vi "Main.vi"(7 "sweep rate, /min":dbl=0.2, 8 "sweep to:":dbl=-0.5, 9 "sweep":T6(radio)=enum."time_sweep") -> ()   [LabVIEW 2017] (continued)
                    n4522 = property on="Down Rate" class="DigNum (strict)"() -> ("Value"=w5909:dbl)  [unwired: 2 in, 2 out]
                    n4523 = property on="lower limit" class="DigNum (strict)"() -> ("Value"=w5910:dbl)  [unwired: 2 in, 2 out]
                    n4524 = property on="sweep to:" class="DigNum (strict)"("Value"=w5910) -> ()  [unwired: 2 in, 2 out]
                    n4525 = property on="sweep rate, /min" class="DigNum (strict)"("Value"=w5909) -> ()  [unwired: 2 in, 2 out]
                  }
                  frame "Sweep Up" {
                    n4526 = property on="Up Rate" class="DigNum (strict)"() -> ("Value"=w5911:dbl)  [unwired: 2 in, 2 out]
                    n4527 = property on="upper limit" class="DigNum (strict)"() -> ("Value"=w5912:dbl)  [unwired: 2 in, 2 out]
                    n4528 = property on="sweep to:" class="DigNum (strict)"("Value"=w5912) -> ()  [unwired: 2 in, 2 out]
                    n4529 = property on="sweep rate, /min" class="DigNum (strict)"("Value"=w5911) -> ()  [unwired: 2 in, 2 out]
                  }
                  frame "True" {
                  }
                }
              }
              frame #3 {
                n4530 = Enqueue Element(queue=w5914, element="Start Sweep") -> ()  [unwired: 2 in, 3 out]
              }
            }
          }
          frame True {
            # "When step values are all finished"
            n4531 = property on="HyperLoop" class="Bool (strict)"() -> ("Value"=w5916:bool)  [unwired: 2 in, 2 out]
            n4532 = property on="Table Index" class="DigNum (strict)"("Value"=0.0 ("Table Index")) -> ()  [unwired: 2 in, 2 out]
            n4533 = case shown="True" w5916 {
              tunnel: w5917 -> [w5923 w5928]
              frame False {
                n4534 = Enqueue Element(queue=w5923, element="Idle") -> ()  [unwired: 2 in, 3 out]
                n4535 = property on="Start Mapping" class="Bool"("DisabledEnum"=T12."Enabled" ("Disabled")) -> ()  [unwired: 2 in, 2 out]
                n4536 = property on="Stop Mapping" class="Bool"("DisabledEnum"=T12."Disabled and Grayed Out" ("Disabled")) -> ()  [unwired: 2 in, 2 out]
                n4537 = property on="Sweep Direction" class="Str"("Value"="Finished!" ("Sweep Direction"), "Text.TextColor"=u32 16711680 ("Text.Text Colors:Text Color")) -> ()  [unwired: 2 in, 2 out]
              }
              frame True {
                n4538 = Enqueue Element(queue=w5928, element="Step to Next HyperLoop Value") -> ()  [unwired: 2 in, 3 out]
                n4539 = property on="HyperLoop Index" class="DigNum (strict)"() -> ("Value"=w5926:dbl)  [unwired: 2 in, 2 out]
                n4540 = property on="Start Mapping" class="Bool"("DisabledEnum"=T12."Enabled" ("Disabled")) -> ()  [unwired: 2 in, 2 out]
                n4541 = property on="Stop Mapping" class="Bool"("DisabledEnum"=T12."Disabled and Grayed Out" ("Disabled")) -> ()  [unwired: 2 in, 2 out]
                n4542 = Increment(x=w5926) -> (x+1=w5927:dbl)
                n4543 = property on="HyperLoop Index" class="DigNum (strict)"("Value"=w5927) -> ()  [unwired: 2 in, 2 out]
                n4544 = property on="Sweep Direction" class="Str"("Value"="Finished!" ("Sweep Direction"), "Text.TextColor"=u32 16711680 ("Text.Text Colors:Text Color")) -> ()  [unwired: 2 in, 2 out]
              }
            }
          }
        }
      }
      frame "Step to Next HyperLoop Value" {
        n4545 = property on="HyperLoop Index" class="DigNum (strict)"() -> ("Value"=w5933:dbl)  [unwired: 2 in, 2 out]
        n4546 = property on="HyperLoop Steps" class="Tbl (strict)"() -> ("Value"=w5932:string[][])  [unwired: 2 in, 2 out]
        n4547 = Equal?(x=w5933, y=0) -> (x = y?=w5944:bool)
        n4548 = case shown="True" w5944 {
          tunnel: w5933 -> [w5952 w5958]
          tunnel: cluster{"Row":i32, "Column":i32} {"Row"=0, "Column"=0} ("Active Cell:Active Cell") -> [w5951 w5957]
          frame False {
            w5953 = 0 ("Column")
            n4549 = Decrement(x=w5952) -> (x-1=w5954:dbl)
            n4550 = Bundle By Name(cluster=w5951, "Row"=w5952, "Column"=w5953) -> (w5950:cluster{"Row":i32, "Column":i32})
            n4551 = Bundle By Name(cluster=w5950, "Row"=w5954, "Column"=w5953) -> (w5948:cluster{"Row":i32, "Column":i32})
            n4552 = property on="HyperLoop Steps" class="Tbl (strict)"("Active Cell"=w5948, "Cell BG Color"=u32 16711680 ("Active Cell:Cell Background Color")) -> ()  [unwired: 2 in, 2 out]
            n4553 = property on="HyperLoop Steps" class="Tbl (strict)"("Active Cell"=w5950, "Cell BG Color"=u32 16776072 ("Active Cell:Cell Background Color")) -> ()  [unwired: 2 in, 2 out]
          }
          frame True {
            n4554 = Bundle By Name(cluster=w5957, "Row"=w5958, "Column"=0) -> (w5956:cluster{"Row":i32, "Column":i32})
            n4555 = property on="HyperLoop Steps" class="Tbl (strict)"("Active Cell"=w5956, "Cell BG Color"=u32 16776072 ("Active Cell:Cell Background Color")) -> ()  [unwired: 2 in, 2 out]
          }
        }
        n4556 = call <vilib>:"Space Constant.vi"() -> ("String"=w5942:string)
        n4557 = Index Array(array=w5932, index (row)=w5933, index (col)=0 ("disabled index (col)")) -> (element=w5941:string)
        n4558 = call <vilib>:"Search and Replace Pattern.vi"("string"=w5941, "regular expression (\"\")"=w5942, "replace string (\"\")"="" ("replace string (\"\")"), "replace all? (F)"=TRUE) -> ("result string"=w5945:string)  [unwired: 1 in, 1 out]
        n4559 = Equal?(x="", y=w5945) -> (x = y?=w5943:bool)
        n4560 = Fract/Exp String To Number(string=w5945) -> (number=w5946:dbl)  [unwired: 3 in, 1 out]
        n4561 = case shown="False" w5943 {
          tunnel: w5946 -> [w5960 _]
          tunnel: w5935 -> [w5961 w6137]
          frame False {
            # "When step values are not finished"
            n4562 = stacked-sequence {
              tunnel: w5960 -> [w5963 _ _]
              tunnel: w5961 -> [_ _ _]
              frame #0 {
                # "1 = 2400 1\n2 = 2400 2\n\n4 = 2636a smua\n5 = 2636a smub\n6 = do not sweep, just time\n7 = iPS, magnetic field \n8 = iTC, temperature"
                # "set next value in the sweep"
                n4563 = property on="step_hyper" class="RadioBtnsControl (strict)"() -> ("Value"=w5962:T9)  [unwired: 2 in, 2 out]
                n4564 = case shown="\"iTC_HyperLoop\"" w5962 {
                  tunnel: w5963 -> [w5965 w5972 _ _ _ w6030 w6094]
                  tunnel: w5963 -> [_ _ w5981 w6007 _ _ _]
                  frame "2400_1_HyperLoop" {
                    # "sweep voltage on 2400 1"
                    n4565 = property on="2400_1_addr_hyper" class="DigNum (strict)"() -> ("Value"=w5964:u8)  [unwired: 2 in, 2 out]
                    n4566 = Number To Fractional String(number=w5965) -> (F-format string=w5970:string)  [unwired: 3 in]
                    n4567 = Concatenate Strings(":INIT:IMM; :SOUR:VOLT:LEV:IMM:AMPL " ("data"), w5970) -> (w5968:string)
                    n4568 = Number To Decimal String(number=w5964) -> (decimal integer string=w5966:string)  [unwired: 1 in]
                    n4569 = GPIB Write(0:w5966, 1:w5968, 2:i16 1 ("mode (0)")) -> ()  [unwired: 2 in, 2 out]
                  }
                  frame "2400_2_HyperLoop" {
                    # "sweep voltage on 2400 2"
                    n4570 = property on="2400_2_addr_hyper" class="DigNum (strict)"() -> ("Value"=w5971:u8)  [unwired: 2 in, 2 out]
                    n4571 = Number To Fractional String(number=w5972) -> (F-format string=w5977:string)  [unwired: 3 in]
                    n4572 = Concatenate Strings(":INIT:IMM; :SOUR:CURR:LEV:IMM:AMPL " ("data"), w5977) -> (w5975:string)
                    n4573 = Number To Decimal String(number=w5971) -> (decimal integer string=w5973:string)  [unwired: 1 in]
                    n4574 = GPIB Write(0:w5973, 1:w5975, 2:i16 1 ("mode (0)")) -> ()  [unwired: 2 in, 2 out]
                  }
                  frame "2636_smua_HyperLoop" {
                    # "sweep voltage on 2636a smua"
                    n4575 = property on="Hyper Channel" class="DigNum (strict)"() -> ("Value"=w5978:dbl)  [unwired: 2 in, 2 out]
                    n4576 = property on="2336A_addr_hyper" class="VISAName"() -> ("Value"=w5979:refnum<visa-resource-name>)  [unwired: 2 in, 2 out]
                    n4577 = property on="Hyper_Mini steps" class="DigNum (strict)"() -> ("Value"=w5980:dbl)  [unwired: 2 in, 2 out]
                    n4578 = Subtract(x=w5981, y=w5978) -> (x-y=w5982:dbl)
                    n4579 = Divide(x=w5982, y=w5980) -> (x/y=w5983:dbl)
                    n4580 = for {
                      N: w5980 -> [_]
                      tunnel: w5978 -> [w5993]
                      tunnel: w5983 -> [w5992]
                      tunnel: w5979 -> [w5989]
                      i -> [w5988]
                      n4581 = Increment(x=w5988) -> (x+1=w5987:i32)
                      n4582 = Multiply(x=w5992, y=w5987) -> (x*y=w5991:dbl)
                      n4583 = Add(x=w5991, y=w5993) -> (x+y=w5984:dbl)
                      n4584 = call "setLevel.vi"("VISA resource name 2"=w5989, "Source"=Source."Voltage", "Channel"=Channel."a", "SourceLevel"=w5984) -> ("VISA resource name"=w5986:refnum<visa-resource-name>)  [unwired: 1 in, 2 out]
                      n4585 = Wait (ms)(milliseconds to wait=u32 12) -> ()  [unwired: 1 out]
                      n4586 = property on="diagonal_hyper" class="Bool (strict)"() -> ("Value"=w5985:bool)  [unwired: 2 in, 2 out]
                      n4587 = property on="Hyper Channel" class="DigNum (strict)"("Value"=w5984) -> ()  [unwired: 2 in, 2 out]
                      n4588 = case shown="True" w5985 {
                        tunnel: w5984 -> [_ w6003]
                        tunnel: w5986 -> [_ w5998]
                        frame False {
                        }
                        frame True {
                          n4589 = property on="Hyper Offset" class="DigNum (strict)"() -> ("Value"=w5996:dbl)  [unwired: 2 in, 2 out]
                          n4590 = property on="Hyper Slope" class="DigNum (strict)"() -> ("Value"=w5997:dbl)  [unwired: 2 in, 2 out]
                          n4591 = Multiply(x=w6003, y=w5997) -> (x*y=w6002:dbl)
                          n4592 = Add(x=w6002, y=w5996) -> (x+y=w5999:dbl)
                          n4593 = call "setLevel.vi"("VISA resource name 2"=w5998, "Source"=Source."Voltage", "Channel"=Channel."b", "SourceLevel"=w5999) -> ()  [unwired: 1 in, 3 out]
                        }
                      }
                    }
                  }
                  frame "2636_smub_HyperLoop" {
                    # "sweep voltage on 2636a smua"
                    n4594 = property on="Hyper Channel" class="DigNum (strict)"() -> ("Value"=w6004:dbl)  [unwired: 2 in, 2 out]
                    n4595 = property on="Hyper_Mini steps" class="DigNum (strict)"() -> ("Value"=w6006:dbl)  [unwired: 2 in, 2 out]
                    n4596 = property on="2336A_addr_hyper" class="VISAName"() -> ("Value"=w6005:refnum<visa-resource-name>)  [unwired: 2 in, 2 out]
                    n4597 = Subtract(x=w6007, y=w6004) -> (x-y=w6008:dbl)
                    n4598 = Divide(x=w6008, y=w6006) -> (x/y=w6009:dbl)
                    n4599 = for {
                      N: w6006 -> [_]
                      tunnel: w6004 -> [w6019]
                      tunnel: w6009 -> [w6018]
                      tunnel: w6005 -> [w6015]
                      i -> [w6014]
                      n4600 = Increment(x=w6014) -> (x+1=w6013:i32)
                      n4601 = Multiply(x=w6018, y=w6013) -> (x*y=w6017:dbl)
                      n4602 = Add(x=w6017, y=w6019) -> (x+y=w6010:dbl)
                      n4603 = property on="diagonal_hyper" class="Bool (strict)"() -> ("Value"=w6011:bool)  [unwired: 2 in, 2 out]
                      n4604 = call "setLevel.vi"("VISA resource name 2"=w6015, "Source"=Source."Voltage", "Channel"=Channel."b", "SourceLevel"=w6010) -> ("VISA resource name"=w6012:refnum<visa-resource-name>)  [unwired: 1 in, 2 out]
                      n4605 = Wait (ms)(milliseconds to wait=u32 12) -> ()  [unwired: 1 out]
                      n4606 = case shown="True" w6011 {
                        tunnel: w6010 -> [_ w6029]
                        tunnel: w6012 -> [_ w6024]
                        frame False {
                        }
                        frame True {
                          n4607 = property on="Hyper Offset" class="DigNum (strict)"() -> ("Value"=w6022:dbl)  [unwired: 2 in, 2 out]
                          n4608 = property on="Hyper Slope" class="DigNum (strict)"() -> ("Value"=w6023:dbl)  [unwired: 2 in, 2 out]
                          n4609 = Multiply(x=w6029, y=w6023) -> (x*y=w6028:dbl)
                          n4610 = Add(x=w6028, y=w6022) -> (x+y=w6025:dbl)
                          n4611 = call "setLevel.vi"("VISA resource name 2"=w6024, "Source"=Source."Voltage", "Channel"=Channel."a", "SourceLevel"=w6025) -> ()  [unwired: 1 in, 3 out]
                        }
                      }
                      n4612 = property on="Hyper Channel" class="DigNum (strict)"("Value"=w6010) -> ()  [unwired: 2 in, 2 out]
                    }
                  }
                  frame "time_HyperLoop", Default {
                    # "do not sweep, just time"
                  }
                  frame "iPS_HyperLoop" {
                    # "step magnetic field"
                    n4613 = stacked-sequence {
                      tunnel: w6030 -> [_ _ _ _ w6045 _ _ _ w6057 _ w6060 _]
                      frame #0 {
                        n4614 = property on="HyperLoop Index" class="DigNum (strict)"() -> ("Value"=w6031:dbl)  [unwired: 2 in, 2 out]
                        n4615 = Equal?(x=w6031, y=0.0) -> (x = y?=w6032:bool)
                        n4616 = case shown="True" w6032 {
                          frame False {
                          }
                          frame True {
                            n4617 = property on="iPS _addr_hyper" class="VISAName"() -> ("Value"=w6036:refnum<visa-resource-name>)  [unwired: 2 in, 2 out]
                            n4618 = property on="Hyper_FieldRate\n(T/min)" class="DigNum (strict)"() -> ("Value"=w6034:dbl)  [unwired: 2 in, 2 out]
                            n4619 = call "iPSset.vi"("Field Rate, T/min"=w6034, "iPSSetCtrl"=iPSsetCtrl."Set Target Field Rate", "VISA resource name"=w6036) -> ("VISA resource name out"=w6035:refnum<visa-resource-name>)  [unwired: 5 in, 3 out]
                            n4620 = property on="iPS _addr_hyper" class="VISAName"("Value"=w6035) -> ()  [unwired: 2 in, 2 out]
                          }
                        }
                      }
                      frame #1 {
                        n4621 = Wait (ms)(milliseconds to wait=u32 500) -> ()  [unwired: 1 out]
                      }
                      frame #2 {
                        n4622 = property on="iPS _addr_hyper" class="VISAName"() -> ("Value"=w6039:refnum<visa-resource-name>)  [unwired: 2 in, 2 out]
                        n4623 = call "iPSset.vi"("iPSSetCtrl"=iPSsetCtrl."Hold", "VISA resource name"=w6039) -> ("VISA resource name out"=w6040:refnum<visa-resource-name>)  [unwired: 6 in, 3 out]
                        n4624 = property on="iPS _addr_hyper" class="VISAName"("Value"=w6040) -> ()  [unwired: 2 in, 2 out]
                      }
                      frame #3 {
                        n4625 = Wait (ms)(milliseconds to wait=u32 500) -> ()  [unwired: 1 out]
                      }
                      frame #4 {
                        n4626 = property on="iPS _addr_hyper" class="VISAName"() -> ("Value"=w6043:refnum<visa-resource-name>)  [unwired: 2 in, 2 out]
                        n4627 = call "iPSset.vi"("Target Field, T"=w6045, "iPSSetCtrl"=iPSsetCtrl."Set Target Field", "VISA resource name"=w6043) -> ("VISA resource name out"=w6044:refnum<visa-resource-name>)  [unwired: 5 in, 3 out]
                        n4628 = property on="iPS _addr_hyper" class="VISAName"("Value"=w6044) -> ()  [unwired: 2 in, 2 out]
                      }
                      frame #5 {
                        n4629 = Wait (ms)(milliseconds to wait=u32 500) -> ()  [unwired: 1 out]
                      }
                      frame #6 {
                        n4630 = property on="iPS _addr_hyper" class="VISAName"() -> ("Value"=w6048:refnum<visa-resource-name>)  [unwired: 2 in, 2 out]
                        n4631 = call "iPSset.vi"("iPSSetCtrl"=iPSsetCtrl."Hold", "VISA resource name"=w6048) -> ("VISA resource name out"=w6049:refnum<visa-resource-name>)  [unwired: 6 in, 3 out]
                        n4632 = property on="iPS _addr_hyper" class="VISAName"("Value"=w6049) -> ()  [unwired: 2 in, 2 out]
                      }
                      frame #7 {
                        n4633 = Wait (ms)(milliseconds to wait=u32 500) -> ()  [unwired: 1 out]
                      }
                      frame #8 {
                        n4634 = Equal To 0?(x=w6057) -> (x = 0?=w6056:bool)
                        n4635 = property on="iPS _addr_hyper" class="VISAName"() -> ("Value"=w6052:refnum<visa-resource-name>)  [unwired: 2 in, 2 out]
                        n4636 = Select(t=iPSsetCtrl."Go to Zero" ("iPSSetCtrl"), s=w6056, f=iPSsetCtrl."Go to Field" ("iPSSetCtrl")) -> (s? t:f=w6053:T18)
                        n4637 = call "iPSset.vi"("iPSSetCtrl"=w6053, "VISA resource name"=w6052) -> ()  [unwired: 6 in, 4 out]
                      }
                      frame #9 {
                        n4638 = Wait (ms)(milliseconds to wait=u32 500) -> ()  [unwired: 1 out]
                      }
                      frame #10 {
                        n4639 = while {
                          tunnel: w6060 -> [w6091]
                          stop <- w6087 stop-if-true
                          n4640 = property on="iPS _addr_hyper" class="VISAName"() -> ("Value"=w6086:refnum<visa-resource-name>)  [unwired: 2 in, 2 out]
                          n4641 = call "iPSread.vi"("iPSreadCtrl"=iPSreadCtrl."MagnetField", "VISA resource name"=w6086) -> ("number"=w6083:dbl, "VISA resource name out"=w6085:refnum<visa-resource-name>)  [unwired: 6 in, 2 out]
                          n4642 = property on="Tolerance_Hyper" class="DigNum (strict)"() -> ("Value"=w6084:dbl)  [unwired: 2 in, 2 out]
                          n4643 = property on="iPS _addr_hyper" class="VISAName"("Value"=w6085) -> ()  [unwired: 2 in, 2 out]
                          n4644 = Wait (ms)(milliseconds to wait=u32 500) -> ()  [unwired: 1 out]
                          n4645 = Subtract(x=w6083, y=w6091) -> (x-y=w6090:dbl)
                          n4646 = Absolute Value(x=w6090) -> (abs(x)=w6089:dbl)
                          n4647 = Less Or Equal?(x=w6089, y=w6084) -> (x <= y?=w6087:bool)
                          n4648 = property on="Hyper Channel" class="DigNum (strict)"("Value"=w6083) -> ()  [unwired: 2 in, 2 out]
                          n4649 = property on="at field_hyper" class="Bool (strict)"("Value"=w6087) -> ()  [unwired: 2 in, 2 out]
                        }
                        n4650 = property on="diagonal_hyper" class="Bool (strict)"() -> ("Value"=w6059:bool)  [unwired: 2 in, 2 out]
                        n4651 = case shown="True" w6059 {
                          tunnel: w6060 -> [_ w6068]
                          frame False {
                          }
                          frame True {
                            n4652 = property on="Channel hyper" class="Enum (strict)"() -> ("Value"=w6062:T2)  [unwired: 2 in, 2 out]
                            n4653 = property on="2336A_addr_hyper" class="VISAName"() -> ("Value"=w6061:refnum<visa-resource-name>)  [unwired: 2 in, 2 out]
                            n4654 = property on="Hyper Offset" class="DigNum (strict)"() -> ("Value"=w6064:dbl)  [unwired: 2 in, 2 out]
                            n4655 = property on="Hyper Slope" class="DigNum (strict)"() -> ("Value"=w6065:dbl)  [unwired: 2 in, 2 out]
                            n4656 = call "SinglePointMeasurement.vi"("Measure"=Measure."Voltage", "Channel"=w6062, "VISA resource name 2"=w6061) -> ("Measuremet"=w6066:dbl)  [unwired: 3 in, 4 out]
                            n4657 = Multiply(x=w6068, y=w6065) -> (x*y=w6072:dbl)
                            n4658 = property on="Hyper_Mini steps" class="DigNum (strict)"() -> ("Value"=w6063:dbl)  [unwired: 2 in, 2 out]
                            n4659 = Add(x=w6072, y=w6064) -> (x+y=w6069:dbl)
                            n4660 = Subtract(x=w6069, y=w6066) -> (x-y=w6070:dbl)
                            n4661 = Divide(x=w6070, y=w6063) -> (x/y=w6071:dbl)
                            n4662 = for {
                              N: w6063 -> [_]
                              tunnel: w6071 -> [w6081]
                              tunnel: w6061 -> [w6078]
                              tunnel: w6066 -> [w6074]
                              i -> [w6076]
                              n4663 = Increment(x=w6076) -> (x+1=w6075:i32)
                              n4664 = Multiply(x=w6081, y=w6075) -> (x*y=w6080:dbl)
                              n4665 = Add(x=w6080, y=w6074) -> (x+y=w6077:dbl)
                              n4666 = property on="Channel 2" class="Enum (strict)"() -> ("Value"=w6073:T2)  [unwired: 2 in, 2 out]
                              n4667 = Wait (ms)(milliseconds to wait=u32 12) -> ()  [unwired: 1 out]
                              n4668 = call "setLevel.vi"("VISA resource name 2"=w6078, "Source"=Source."Voltage", "Channel"=w6073, "SourceLevel"=w6077) -> ()  [unwired: 1 in, 3 out]
                            }
                          }
                        }
                      }
                      frame #11 {
                        n4669 = Wait (ms)(milliseconds to wait=u32 500) -> ()  [unwired: 1 out]
                      }
                    }
                  }
                  frame "iTC_HyperLoop" {
                    # "step temperature"
                    n4670 = stacked-sequence {
                      tunnel: w6094 -> [w6102 w6106 w6112]
                      frame #0 {
                        n4671 = property on="iTC_addr_hyper" class="VISAName"() -> ("Value"=w6096:refnum<visa-resource-name>)  [unwired: 2 in, 2 out]
                        n4672 = Decrement(x=w6102) -> (x-1=w6099:dbl)
                        n4673 = Less Or Equal To 0?(x=w6099) -> (x <= 0?=w6101:bool)
                        n4674 = Select(t=0.0, s=w6101, f=w6099) -> (s? t:f=w6098:dbl)
                        n4675 = call "iTCset.vi"("Set Point"=w6098, "iTCSetCtrl"=iTCsetCtrl."Set VTI Temp", "VISA resource name"=w6096) -> ("VISA resource name out"=w6095:refnum<visa-resource-name>)  [unwired: 5 in, 3 out]
                        n4676 = Wait (ms)(milliseconds to wait=u32 200) -> ()  [unwired: 1 out]
                        n4677 = property on="iTC_addr_hyper" class="VISAName"("Value"=w6095) -> ()  [unwired: 2 in, 2 out]
                      }
                      frame #1 {
                        n4678 = property on="iTC_addr_hyper" class="VISAName"() -> ("Value"=w6104:refnum<visa-resource-name>)  [unwired: 2 in, 2 out]
                        n4679 = Less Or Equal To 0?(x=w6106) -> (x <= 0?=w6110:bool)
                        n4680 = Select(t=0.0, s=w6110, f=w6106) -> (s? t:f=w6108:dbl)
                        n4681 = call "iTCset.vi"("Set Point"=w6108, "iTCSetCtrl"=iTCsetCtrl."Set Sample Temp", "VISA resource name"=w6104) -> ("VISA resource name out"=w6105:refnum<visa-resource-name>)  [unwired: 5 in, 3 out]
                        n4682 = property on="iTC_addr_hyper" class="VISAName"("Value"=w6105) -> ()  [unwired: 2 in, 2 out]
                        n4683 = Wait (ms)(milliseconds to wait=u32 200) -> ()  [unwired: 1 out]
                      }
                      frame #2 {
                        n4684 = while {
                          tunnel: w6112 -> [w6119]
                          stop <- w6115 stop-if-true
                          n4685 = property on="iTC_addr_hyper" class="VISAName"() -> ("Value"=w6116:refnum<visa-resource-name>)  [unwired: 2 in, 2 out]
                          n4686 = property on="Tolerance_Hyper" class="DigNum (strict)"() -> ("Value"=w6114:dbl)  [unwired: 2 in, 2 out]
                          n4687 = call "iTCread.vi"("VISA resource name"=w6116, "iTCreadCtrl"=iTCreadCtrl."Sample Temp") -> ("number"=w6113:dbl)  [unwired: 5 in, 3 out]
                          n4688 = Subtract(x=w6113, y=w6119) -> (x-y=w6118:dbl)
                          n4689 = Absolute Value(x=w6118) -> (abs(x)=w6117:dbl)
                          n4690 = property on="Hyper Channel" class="DigNum (strict)"("Value"=w6113) -> ()  [unwired: 2 in, 2 out]
                          n4691 = Less?(x=w6117, y=w6114) -> (x < y?=w6115:bool)
                          n4692 = property on="at field_hyper" class="Bool (strict)"("Value"=w6115) -> ()  [unwired: 2 in, 2 out]
                        }
                      }
                    }
                  }
                }
              }
              frame #1 {
                # "Set current hyper channel and wait expected time"
                n4693 = property on="Current Hyper Value" class="DigNum (strict)"() -> ("Value"=w6122:dbl)  [unwired: 2 in, 2 out]
                n4694 = property on="Wait Between Hyper" class="DigNum (strict)"() -> ("Value"=w6121:i32)  [unwired: 2 in, 2 out]
                n4695 = property on="Hyper Channel" class="DigNum (strict)"("Value"=w6122) -> ()  [unwired: 2 in, 2 out]
                n4696 = Multiply(x=w6121, y=1000) -> (x*y=w6123:i32)
                n4697 = Wait (ms)(milliseconds to wait=w6123) -> ()  [unwired: 1 out]
              }
              frame #2 {
                n4698 = stacked-sequence {
                  frame #0 {
                    # "Check if need to swap step direction"
                    n4699 = property on="SwapStepDirection" class="Bool (strict)"() -> ("Value"=w6125:bool)  [unwired: 2 in, 2 out]
                    n4700 = case shown="True" w6125 {
                      frame False {
                      }
                      frame True {
                        n4701 = stacked-sequence {
                          frame #0 {
                            n4702 = property on="HyperLoop Index" class="DigNum (strict)"() -> ("Value"=w6127:dbl)  [unwired: 2 in, 2 out]
                            n4703 = Equal To 0?(x=w6127) -> (x = 0?=w6126:bool)
                            n4704 = case shown="False" w6126 {
                              frame False {
                                n4705 = property on="to" class="DigNum (strict)"() -> ("Value"=w6131:dbl)  [unwired: 2 in, 2 out]
                                n4706 = property on="from" class="DigNum (strict)"() -> ("Value"=w6130:dbl)  [unwired: 2 in, 2 out]
                                n4707 = Swap Values(12:w6131, 14:w6130) -> (1:w6129:dbl, 3:w6128:dbl)  [unwired: 1 in]
                                n4708 = property on="from" class="DigNum (strict)"("Value"=w6128) -> ()  [unwired: 2 in, 2 out]
                                n4709 = property on="to" class="DigNum (strict)"("Value"=w6129) -> ()  [unwired: 2 in, 2 out]
                              }
                              frame True {
                              }
                            }
                          }
                          frame #1 {
                            n4710 = property on="HyperLoop Index" class="DigNum (strict)"() -> ("Value"=w6133:dbl)  [unwired: 2 in, 2 out]
                            n4711 = Equal To 0?(x=w6133) -> (x = 0?=w6132:bool)
                            n4712 = case shown="False" w6132 {
                              frame False {
                                n4713 = property on="Hidden_HyperLoop_Swap" class="Bool (strict)"() -> ("Value"=w6134:bool)  [unwired: 2 in, 2 out]
                                n4714 = property on="Hidden_HyperLoop_Swap" class="Bool (strict)"("Val(Sgnl)"=w6134) -> ()  [unwired: 2 in, 2 out]
                              }
                              frame True {
                              }
                            }
                          }
                        }
                      }
                    }
                  }
                  frame #1 {
                    # "Trigger \"start mapping\" event"
                    n4715 = property on="HyperLoop Hidden" class="Bool (strict)"() -> ("Value"=w6135:bool)  [unwired: 2 in, 2 out]
                    n4716 = property on="HyperLoop Hidden" class="Bool (strict)"("Val(Sgnl)"=w6135) -> ()  [unwired: 2 in, 2 out]
                  }
                }
              }
            }
            n4717 = property on="Current Hyper Value" class="DigNum (strict)"("Value"=w5960) -> ()  [unwired: 2 in, 2 out]
          }
          frame True {
            # "When step values are all finished"
            n4718 = property on="SuperHyper" class="Bool (strict)"() -> ("Value"=w6136:bool)  [unwired: 2 in, 2 out]
            n4719 = case shown="True" w6136 {
              tunnel: w6137 -> [w6143 w6151]
              frame False {
                n4720 = Enqueue Element(queue=w6143, element="Idle") -> ()  [unwired: 2 in, 3 out]
                n4721 = property on="Stop HyperLoop" class="Bool"("DisabledEnum"=T12."Disabled and Grayed Out" ("Disabled")) -> ()  [unwired: 2 in, 2 out]
                n4722 = property on="Start HyperLoop" class="Bool"("DisabledEnum"=T12."Enabled" ("Disabled")) -> ()  [unwired: 2 in, 2 out]
                n4723 = property on="Sweep Direction 2" class="Str"("Value"="Finished!" ("Sweep Direction"), "Text.TextColor"=u32 16711680 ("Text.Text Colors:Text Color")) -> ()  [unwired: 2 in, 2 out]
              }
              frame True {
                n4724 = Enqueue Element(queue=w6151, element="Step to Next SuperHyper Value") -> ()  [unwired: 2 in, 3 out]
                n4725 = property on="SuperHyper_Index" class="DigNum (strict)"() -> ("Value"=w6149:dbl)  [unwired: 2 in, 2 out]
                n4726 = Increment(x=w6149) -> (x+1=w6148:dbl)
                n4727 = property on="Start HyperLoop" class="Bool"("DisabledEnum"=T12."Enabled" ("Disabled")) -> ()  [unwired: 2 in, 2 out]
                n4728 = property on="Stop HyperLoop" class="Bool"("DisabledEnum"=T12."Disabled and Grayed Out" ("Disabled")) -> ()  [unwired: 2 in, 2 out]
                n4729 = property on="SuperHyper_Index" class="DigNum (strict)"("Value"=w6148) -> ()  [unwired: 2 in, 2 out]
                n4730 = property on="Sweep Direction_Hyper" class="Str"("Value"="Finished!" ("Sweep Direction"), "Text.TextColor"=u32 16711680 ("Text.Text Colors:Text Color")) -> ()  [unwired: 2 in, 2 out]
              }
            }
          }
        }
      }
      frame "Step to Next SuperHyper Value" {
        n4731 = property on="SuperHyper_Index" class="DigNum (strict)"() -> ("Value"=w6152:dbl)  [unwired: 2 in, 2 out]
        n4732 = property on="SuperHyper Steps" class="Tbl (strict)"() -> ("Value"=w6153:string[][])  [unwired: 2 in, 2 out]
        n4733 = Equal?(x=w6152, y=0) -> (x = y?=w6164:bool)
        n4734 = case shown="False" w6164 {
          tunnel: w6152 -> [w6172 w6178]
          tunnel: cluster{"Row":i32, "Column":i32} {"Row"=0, "Column"=0} ("Active Cell:Active Cell") -> [w6171 w6177]
          frame False {
            w6173 = 0 ("Column")
            n4735 = Decrement(x=w6172) -> (x-1=w6174:dbl)
            n4736 = Bundle By Name(cluster=w6171, "Row"=w6172, "Column"=w6173) -> (w6170:cluster{"Row":i32, "Column":i32})
            n4737 = Bundle By Name(cluster=w6170, "Row"=w6174, "Column"=w6173) -> (w6168:cluster{"Row":i32, "Column":i32})
            n4738 = property on="SuperHyper Steps" class="Tbl (strict)"("Active Cell"=w6170, "Cell BG Color"=u32 16776072 ("Active Cell:Cell Background Color")) -> ()  [unwired: 2 in, 2 out]
            n4739 = property on="SuperHyper Steps" class="Tbl (strict)"("Active Cell"=w6168, "Cell BG Color"=u32 16711680 ("Active Cell:Cell Background Color")) -> ()  [unwired: 2 in, 2 out]
          }
          frame True {
            n4740 = Bundle By Name(cluster=w6177, "Row"=w6178, "Column"=0) -> (w6176:cluster{"Row":i32, "Column":i32})
            n4741 = property on="SuperHyper Steps" class="Tbl (strict)"("Active Cell"=w6176, "Cell BG Color"=u32 16776072 ("Active Cell:Cell Background Color")) -> ()  [unwired: 2 in, 2 out]
          }
        }
        n4742 = call <vilib>:"Space Constant.vi"() -> ("String"=w6162:string)
        n4743 = Index Array(array=w6153, index (row)=w6152, index (col)=0 ("disabled index (col)")) -> (element=w6161:string)
        n4744 = call <vilib>:"Search and Replace Pattern.vi"("string"=w6161, "regular expression (\"\")"=w6162, "replace string (\"\")"="" ("replace string (\"\")"), "replace all? (F)"=TRUE) -> ("result string"=w6165:string)  [unwired: 1 in, 1 out]
        n4745 = Equal?(x="", y=w6165) -> (x = y?=w6163:bool)
        n4746 = Fract/Exp String To Number(string=w6165) -> (number=w6166:dbl)  [unwired: 3 in, 1 out]
        n4747 = case shown="False" w6163 {
          tunnel: w6166 -> [w6180 _]
          tunnel: w6155 -> [w6181 w6359]
          frame False {
            # "When step values are not finished"
            n4748 = stacked-sequence {
              tunnel: w6180 -> [w6183 _ _ _]
              tunnel: w6181 -> [_ _ _ _]
              frame #0 {
                # "1 = 2400 1\n2 = 2400 2\n\n4 = 2636a smua\n5 = 2636a smub\n6 = do not sweep, just time\n7 = iPS, magnetic field \n8 = iTC, temperature"
                # "set next value in the sweep"
                n4749 = property on="step_super" class="RadioBtnsControl (strict)"() -> ("Value"=w6182:T10)  [unwired: 2 in, 2 out]
                n4750 = case shown="\"2636_smub_SuperHyper\"" w6182 {
                  tunnel: w6183 -> [w6185 w6192 _ _ _ w6250 w6314]
                  tunnel: w6183 -> [_ _ w6201 w6227 _ _ _]
                  frame "2400_1_SuperHyper" {
                    # "sweep voltage on 2400 1"
                    n4751 = property on="2400_1_addr_superhyper" class="DigNum (strict)"() -> ("Value"=w6184:u8)  [unwired: 2 in, 2 out]
                    n4752 = Number To Fractional String(number=w6185) -> (F-format string=w6190:string)  [unwired: 3 in]
                    n4753 = Concatenate Strings(":INIT:IMM; :SOUR:VOLT:LEV:IMM:AMPL " ("data"), w6190) -> (w6188:string)
                    n4754 = Number To Decimal String(number=w6184) -> (decimal integer string=w6186:string)  [unwired: 1 in]
                    n4755 = GPIB Write(0:w6186, 1:w6188, 2:i16 1 ("mode (0)")) -> ()  [unwired: 2 in, 2 out]
                  }
                  frame "2400_2_SuperHyper" {
                    # "sweep voltage on 2400 2"
                    n4756 = property on="2400_2_addr_superhyper" class="DigNum (strict)"() -> ("Value"=w6191:u8)  [unwired: 2 in, 2 out]
                    n4757 = Number To Fractional String(number=w6192) -> (F-format string=w6197:string)  [unwired: 3 in]
                    n4758 = Concatenate Strings(":INIT:IMM; :SOUR:CURR:LEV:IMM:AMPL " ("data"), w6197) -> (w6195:string)
                    n4759 = Number To Decimal String(number=w6191) -> (decimal integer string=w6193:string)  [unwired: 1 in]
                    n4760 = GPIB Write(0:w6193, 1:w6195, 2:i16 1 ("mode (0)")) -> ()  [unwired: 2 in, 2 out]
                  }
                  frame "2636_smua_SuperHyper" {
                    # "sweep voltage on 2636a smua"
                    n4761 = property on="SuperHyper" class="DigNum (strict)"() -> ("Value"=w6198:dbl)  [unwired: 2 in, 2 out]
                    n4762 = property on="Super_ministeps" class="DigNum (strict)"() -> ("Value"=w6199:dbl)  [unwired: 2 in, 2 out]
                    n4763 = property on="2336A_addr_superhyper" class="VISAName"() -> ("Value"=w6200:refnum<visa-resource-name>)  [unwired: 2 in, 2 out]
                    n4764 = Subtract(x=w6201, y=w6198) -> (x-y=w6202:dbl)
                    n4765 = Divide(x=w6202, y=w6199) -> (x/y=w6203:dbl)
                    n4766 = for {
                      N: w6199 -> [_]
                      tunnel: w6198 -> [w6213]
                      tunnel: w6203 -> [w6212]
                      tunnel: w6200 -> [w6209]
                      i -> [w6208]
                      n4767 = Increment(x=w6208) -> (x+1=w6207:i32)
                      n4768 = Multiply(x=w6212, y=w6207) -> (x*y=w6211:dbl)
                      n4769 = Add(x=w6211, y=w6213) -> (x+y=w6204:dbl)
                      n4770 = property on="diagona_super" class="Bool (strict)"() -> ("Value"=w6205:bool)  [unwired: 2 in, 2 out]
                      n4771 = call "setLevel.vi"("VISA resource name 2"=w6209, "Source"=Source."Voltage", "Channel"=Channel."a", "SourceLevel"=w6204) -> ("VISA resource name"=w6206:refnum<visa-resource-name>)  [unwired: 1 in, 2 out]
                      n4772 = Wait (ms)(milliseconds to wait=u32 12) -> ()  [unwired: 1 out]
                      n4773 = case shown="True" w6205 {
                        tunnel: w6204 -> [_ w6223]
                        tunnel: w6206 -> [_ w6218]
                        frame False {
                        }
                        frame True {
                          n4774 = property on="Slope_super" class="DigNum (strict)"() -> ("Value"=w6217:dbl)  [unwired: 2 in, 2 out]
                          n4775 = property on="Offset_super" class="DigNum (strict)"() -> ("Value"=w6216:dbl)  [unwired: 2 in, 2 out]
                          n4776 = Multiply(x=w6223, y=w6217) -> (x*y=w6222:dbl)
                          n4777 = Add(x=w6222, y=w6216) -> (x+y=w6219:dbl)
                          n4778 = call "setLevel.vi"("VISA resource name 2"=w6218, "Source"=Source."Voltage", "Channel"=Channel."b", "SourceLevel"=w6219) -> ()  [unwired: 1 in, 3 out]
                        }
                      }
                      n4779 = property on="SuperHyper" class="DigNum (strict)"("Value"=w6204) -> ()  [unwired: 2 in, 2 out]
                    }
                  }
                  frame "2636_smub_SuperHyper" {
                    # "sweep voltage on 2636a smua"
                    n4780 = property on="SuperHyper" class="DigNum (strict)"() -> ("Value"=w6224:dbl)  [unwired: 2 in, 2 out]
                    n4781 = property on="Super_ministeps" class="DigNum (strict)"() -> ("Value"=w6225:dbl)  [unwired: 2 in, 2 out]
                    n4782 = property on="2336A_addr_superhyper" class="VISAName"() -> ("Value"=w6226:refnum<visa-resource-name>)  [unwired: 2 in, 2 out]
                    n4783 = Subtract(x=w6227, y=w6224) -> (x-y=w6228:dbl)
                    n4784 = Divide(x=w6228, y=w6225) -> (x/y=w6229:dbl)
                    n4785 = for {
                      N: w6225 -> [_]
                      tunnel: w6224 -> [w6239]
                      tunnel: w6229 -> [w6238]
                      tunnel: w6226 -> [w6235]
                      i -> [w6234]
                      n4786 = Increment(x=w6234) -> (x+1=w6233:i32)
                      n4787 = Multiply(x=w6238, y=w6233) -> (x*y=w6237:dbl)
                      n4788 = Add(x=w6237, y=w6239) -> (x+y=w6230:dbl)
                      n4789 = property on="diagona_super" class="Bool (strict)"() -> ("Value"=w6231:bool)  [unwired: 2 in, 2 out]
                      n4790 = call "setLevel.vi"("VISA resource name 2"=w6235, "Source"=Source."Voltage", "Channel"=Channel."b", "SourceLevel"=w6230) -> ("VISA resource name"=w6232:refnum<visa-resource-name>)  [unwired: 1 in, 2 out]
                      n4791 = Wait (ms)(milliseconds to wait=u32 12) -> ()  [unwired: 1 out]
                      n4792 = case shown="True" w6231 {
                        tunnel: w6230 -> [_ w6249]
                        tunnel: w6232 -> [_ w6244]
                        frame False {
                        }
                        frame True {
                          n4793 = property on="Offset_super" class="DigNum (strict)"() -> ("Value"=w6242:dbl)  [unwired: 2 in, 2 out]
                          n4794 = property on="Slope_super" class="DigNum (strict)"() -> ("Value"=w6243:dbl)  [unwired: 2 in, 2 out]
                          n4795 = Multiply(x=w6249, y=w6243) -> (x*y=w6248:dbl)
                          n4796 = Add(x=w6248, y=w6242) -> (x+y=w6245:dbl)
                          n4797 = call "setLevel.vi"("VISA resource name 2"=w6244, "Source"=Source."Voltage", "Channel"=Channel."a", "SourceLevel"=w6245) -> ()  [unwired: 1 in, 3 out]
                        }
                      }
                      n4798 = property on="SuperHyper" class="DigNum (strict)"("Value"=w6230) -> ()  [unwired: 2 in, 2 out]
                    }
                  }
                  frame "time_SuperHyper", Default {
                    # "do not sweep, just time"
                  }
                  frame "iPS_SuperHyper" {
                    # "step magnetic field"
                    n4799 = stacked-sequence {
                      tunnel: w6250 -> [_ _ _ _ w6265 _ _ _ w6277 _ w6280 _]
                      frame #0 {
                        n4800 = property on="SuperHyper_Index" class="DigNum (strict)"() -> ("Value"=w6251:dbl)  [unwired: 2 in, 2 out]
                        n4801 = Equal?(x=w6251, y=0.0) -> (x = y?=w6252:bool)
                        n4802 = case shown="True" w6252 {
                          frame False {
                          }
                          frame True {
                            n4803 = property on="iPS _addr_superhyper" class="VISAName"() -> ("Value"=w6256:refnum<visa-resource-name>)  [unwired: 2 in, 2 out]
                            n4804 = property on="Super_FieldRate\n(T/min)" class="DigNum (strict)"() -> ("Value"=w6255:dbl)  [unwired: 2 in, 2 out]
                            n4805 = call "iPSset.vi"("Field Rate, T/min"=w6255, "iPSSetCtrl"=iPSsetCtrl."Set Target Field Rate", "VISA resource name"=w6256) -> ("VISA resource name out"=w6254:refnum<visa-resource-name>)  [unwired: 5 in, 3 out]
                            n4806 = property on="iPS _addr_superhyper" class="VISAName"("Value"=w6254) -> ()  [unwired: 2 in, 2 out]
                          }
                        }
                      }
                      frame #1 {
                        n4807 = Wait (ms)(milliseconds to wait=u32 500) -> ()  [unwired: 1 out]
                      }
                      frame #2 {
                        n4808 = property on="iPS _addr_superhyper" class="VISAName"() -> ("Value"=w6260:refnum<visa-resource-name>)  [unwired: 2 in, 2 out]
                        n4809 = call "iPSset.vi"("iPSSetCtrl"=iPSsetCtrl."Hold", "VISA resource name"=w6260) -> ("VISA resource name out"=w6259:refnum<visa-resource-name>)  [unwired: 6 in, 3 out]
                        n4810 = property on="iPS _addr_superhyper" class="VISAName"("Value"=w6259) -> ()  [unwired: 2 in, 2 out]
                      }
                      frame #3 {
                        n4811 = Wait (ms)(milliseconds to wait=u32 500) -> ()  [unwired: 1 out]
                      }
                      frame #4 {
                        n4812 = property on="iPS _addr_superhyper" class="VISAName"() -> ("Value"=w6264:refnum<visa-resource-name>)  [unwired: 2 in, 2 out]
                        n4813 = call "iPSset.vi"("Target Field, T"=w6265, "iPSSetCtrl"=iPSsetCtrl."Set Target Field", "VISA resource name"=w6264) -> ("VISA resource name out"=w6263:refnum<visa-resource-name>)  [unwired: 5 in, 3 out]
                        n4814 = property on="iPS _addr_superhyper" class="VISAName"("Value"=w6263) -> ()  [unwired: 2 in, 2 out]
                      }
                      frame #5 {
                        n4815 = Wait (ms)(milliseconds to wait=u32 500) -> ()  [unwired: 1 out]
                      }
                      frame #6 {
                        n4816 = property on="iPS _addr_superhyper" class="VISAName"() -> ("Value"=w6268:refnum<visa-resource-name>)  [unwired: 2 in, 2 out]
                        n4817 = call "iPSset.vi"("iPSSetCtrl"=iPSsetCtrl."Hold", "VISA resource name"=w6268) -> ("VISA resource name out"=w6269:refnum<visa-resource-name>)  [unwired: 6 in, 3 out]
                        n4818 = property on="iPS _addr_superhyper" class="VISAName"("Value"=w6269) -> ()  [unwired: 2 in, 2 out]
                      }
                      frame #7 {
                        n4819 = Wait (ms)(milliseconds to wait=u32 500) -> ()  [unwired: 1 out]
                      }
                      frame #8 {
                        n4820 = Equal To 0?(x=w6277) -> (x = 0?=w6276:bool)
                        n4821 = property on="iPS _addr_superhyper" class="VISAName"() -> ("Value"=w6272:refnum<visa-resource-name>)  [unwired: 2 in, 2 out]
                        n4822 = Select(t=iPSsetCtrl."Go to Zero" ("iPSSetCtrl"), s=w6276, f=iPSsetCtrl."Go to Field" ("iPSSetCtrl")) -> (s? t:f=w6273:T18)
                        n4823 = call "iPSset.vi"("iPSSetCtrl"=w6273, "VISA resource name"=w6272) -> ()  [unwired: 6 in, 4 out]
                      }
                      frame #9 {
                        n4824 = Wait (ms)(milliseconds to wait=u32 500) -> ()  [unwired: 1 out]
                      }
                      frame #10 {
                        n4825 = while {
                          tunnel: w6280 -> [w6311]
                          stop <- w6304 stop-if-true
                          n4826 = property on="iPS _addr_superhyper" class="VISAName"() -> ("Value"=w6307:refnum<visa-resource-name>)  [unwired: 2 in, 2 out]
                          n4827 = call "iPSread.vi"("iPSreadCtrl"=iPSreadCtrl."MagnetField", "VISA resource name"=w6307) -> ("number"=w6305:dbl, "VISA resource name out"=w6306:refnum<visa-resource-name>)  [unwired: 6 in, 2 out]
                          n4828 = property on="Tolerance_super" class="DigNum (strict)"() -> ("Value"=w6303:dbl)  [unwired: 2 in, 2 out]
                          n4829 = Wait (ms)(milliseconds to wait=u32 500) -> ()  [unwired: 1 out]
                          n4830 = Subtract(x=w6305, y=w6311) -> (x-y=w6310:dbl)
                          n4831 = property on="iPS _addr_superhyper" class="VISAName"("Value"=w6306) -> ()  [unwired: 2 in, 2 out]
                          n4832 = Absolute Value(x=w6310) -> (abs(x)=w6309:dbl)
                          n4833 = Less Or Equal?(x=w6309, y=w6303) -> (x <= y?=w6304:bool)
                          n4834 = property on="SuperHyper" class="DigNum (strict)"("Value"=w6305) -> ()  [unwired: 2 in, 2 out]
                          n4835 = property on="at field_super" class="Bool (strict)"("Value"=w6304) -> ()  [unwired: 2 in, 2 out]
                        }
                        n4836 = property on="diagona_super" class="Bool (strict)"() -> ("Value"=w6279:bool)  [unwired: 2 in, 2 out]
                        n4837 = case shown="True" w6279 {
                          tunnel: w6280 -> [_ w6288]
                          frame False {
                          }
                          frame True {
                            n4838 = property on="Channel" class="Enum (strict)"() -> ("Value"=w6281:T2)  [unwired: 2 in, 2 out]
                            n4839 = property on="Offset_super" class="DigNum (strict)"() -> ("Value"=w6284:dbl)  [unwired: 2 in, 2 out]
                            n4840 = property on="2336A_addr_super" class="VISAName"() -> ("Value"=w6282:refnum<visa-resource-name>)  [unwired: 2 in, 2 out]
                            n4841 = property on="Slope_super" class="DigNum (strict)"() -> ("Value"=w6285:dbl)  [unwired: 2 in, 2 out]
                            n4842 = call "SinglePointMeasurement.vi"("Measure"=Measure."Voltage", "Channel"=w6281, "VISA resource name 2"=w6282) -> ("Measuremet"=w6286:dbl)  [unwired: 3 in, 4 out]
                            n4843 = Multiply(x=w6288, y=w6285) -> (x*y=w6292:dbl)
                            n4844 = property on="Super_ministeps" class="DigNum (strict)"() -> ("Value"=w6283:dbl)  [unwired: 2 in, 2 out]
                            n4845 = Add(x=w6292, y=w6284) -> (x+y=w6289:dbl)
                            n4846 = Subtract(x=w6289, y=w6286) -> (x-y=w6290:dbl)
                            n4847 = Divide(x=w6290, y=w6283) -> (x/y=w6291:dbl)
                            n4848 = for {
                              N: w6283 -> [_]
                              tunnel: w6291 -> [w6301]
                              tunnel: w6282 -> [w6298]
                              tunnel: w6286 -> [w6294]
                              i -> [w6296]
                              n4849 = Increment(x=w6296) -> (x+1=w6295:i32)
                              n4850 = Multiply(x=w6301, y=w6295) -> (x*y=w6300:dbl)
                              n4851 = Add(x=w6300, y=w6294) -> (x+y=w6297:dbl)
                              n4852 = property on="Channel 2" class="Enum (strict)"() -> ("Value"=w6293:T2)  [unwired: 2 in, 2 out]
                              n4853 = Wait (ms)(milliseconds to wait=u32 12) -> ()  [unwired: 1 out]
                              n4854 = call "setLevel.vi"("VISA resource name 2"=w6298, "Source"=Source."Voltage", "Channel"=w6293, "SourceLevel"=w6297) -> ()  [unwired: 1 in, 3 out]
                            }
                          }
                        }
                      }
                      frame #11 {
                        n4855 = Wait (ms)(milliseconds to wait=u32 500) -> ()  [unwired: 1 out]
                      }
                    }
                  }
                  frame "iTC_SuperHyper" {
                    # "step temperature"
                    n4856 = stacked-sequence {
                      tunnel: w6314 -> [w6322 w6326 w6332]
                      frame #0 {
                        n4857 = Decrement(x=w6322) -> (x-1=w6319:dbl)
                        n4858 = property on="iTC_addr_super" class="VISAName"() -> ("Value"=w6316:refnum<visa-resource-name>)  [unwired: 2 in, 2 out]
                        n4859 = Less Or Equal To 0?(x=w6319) -> (x <= 0?=w6321:bool)
                        n4860 = Select(t=0.0, s=w6321, f=w6319) -> (s? t:f=w6318:dbl)
                        n4861 = call "iTCset.vi"("Set Point"=w6318, "iTCSetCtrl"=iTCsetCtrl."Set VTI Temp", "VISA resource name"=w6316) -> ("VISA resource name out"=w6315:refnum<visa-resource-name>)  [unwired: 5 in, 3 out]
                        n4862 = Wait (ms)(milliseconds to wait=u32 200) -> ()  [unwired: 1 out]
                        n4863 = property on="iTC_addr_super" class="VISAName"("Value"=w6315) -> ()  [unwired: 2 in, 2 out]
                      }
                      frame #1 {
                        n4864 = property on="iTC_addr_super" class="VISAName"() -> ("Value"=w6325:refnum<visa-resource-name>)  [unwired: 2 in, 2 out]
                        n4865 = Less Or Equal To 0?(x=w6326) -> (x <= 0?=w6330:bool)
                        n4866 = Select(t=0.0, s=w6330, f=w6326) -> (s? t:f=w6328:dbl)
                        n4867 = call "iTCset.vi"("Set Point"=w6328, "iTCSetCtrl"=iTCsetCtrl."Set Sample Temp", "VISA resource name"=w6325) -> ("VISA resource name out"=w6324:refnum<visa-resource-name>)  [unwired: 5 in, 3 out]
                        n4868 = Wait (ms)(milliseconds to wait=u32 200) -> ()  [unwired: 1 out]
                        n4869 = property on="iTC_addr_super" class="VISAName"("Value"=w6324) -> ()  [unwired: 2 in, 2 out]
                      }
                      frame #2 {
                        n4870 = while {
                          tunnel: w6332 -> [w6339]
                          stop <- w6333 stop-if-true
                          n4871 = property on="iTC_addr_super" class="VISAName"() -> ("Value"=w6336:refnum<visa-resource-name>)  [unwired: 2 in, 2 out]
                          n4872 = property on="Tolerance_super" class="DigNum (strict)"() -> ("Value"=w6334:dbl)  [unwired: 2 in, 2 out]
                          n4873 = call "iTCread.vi"("VISA resource name"=w6336, "iTCreadCtrl"=iTCreadCtrl."Sample Temp") -> ("number"=w6335:dbl)  [unwired: 5 in, 3 out]
                          n4874 = Subtract(x=w6335, y=w6339) -> (x-y=w6338:dbl)
                          n4875 = Absolute Value(x=w6338) -> (abs(x)=w6337:dbl)
                          n4876 = property on="SuperHyper" class="DigNum (strict)"("Value"=w6335) -> ()  [unwired: 2 in, 2 out]
                          n4877 = Less?(x=w6337, y=w6334) -> (x < y?=w6333:bool)
                          n4878 = property on="at field_super" class="Bool (strict)"("Value"=w6333) -> ()  [unwired: 2 in, 2 out]
                        }
                      }
                    }
                  }
                }
              }
              frame #1 {
                # "Set current hyper channel and wait expected time"
                n4879 = property on="Current SuperHyper Value" class="DigNum (strict)"() -> ("Value"=w6342:dbl)  [unwired: 2 in, 2 out]
                n4880 = property on="Wait Btwn SuperHyper" class="DigNum (strict)"() -> ("Value"=w6341:i32)  [unwired: 2 in, 2 out]
                n4881 = Multiply(x=w6341, y=1000) -> (x*y=w6343:i32)
                n4882 = property on="SuperHyper" class="DigNum (strict)"("Value"=w6342) -> ()  [unwired: 2 in, 2 out]
                n4883 = Wait (ms)(milliseconds to wait=w6343) -> ()  [unwired: 1 out]
              }
              frame #2 {
                # "Check if need to swap step direction"
                n4884 = property on="SwapHyperDirection" class="Bool (strict)"() -> ("Value"=w6345:bool)  [unwired: 2 in, 2 out]
                n4885 = case shown="True" w6345 {
                  frame False {
                  }
                  frame True {
                    n4886 = stacked-sequence {
                      frame #0 {
                        n4887 = property on="SuperHyper_Index" class="DigNum (strict)"() -> ("Value"=w6346:dbl)  [unwired: 2 in, 2 out]
                        n4888 = Equal To 0?(x=w6346) -> (x = 0?=w6347:bool)
                        n4889 = case shown="False" w6347 {
                          frame False {
                            n4890 = property on="from" class="DigNum (strict)"() -> ("Value"=w6351:dbl)  [unwired: 2 in, 2 out]
                            n4891 = property on="to" class="DigNum (strict)"() -> ("Value"=w6349:dbl)  [unwired: 2 in, 2 out]
                            n4892 = Swap Values(12:w6349, 14:w6351) -> (1:w6348:dbl, 3:w6350:dbl)  [unwired: 1 in]
                            n4893 = property on="from" class="DigNum (strict)"("Value"=w6350) -> ()  [unwired: 2 in, 2 out]
                            n4894 = property on="to" class="DigNum (strict)"("Value"=w6348) -> ()  [unwired: 2 in, 2 out]
                          }
                          frame True {
                          }
                        }
                      }
                      frame #1 {
                        n4895 = property on="Hidden_super_Swap" class="Bool (strict)"() -> ("Value"=w6352:bool)  [unwired: 2 in, 2 out]
                        n4896 = property on="Hidden_super_Swap" class="Bool (strict)"("Val(Sgnl)"=w6352) -> ()  [unwired: 2 in, 2 out]
                      }
                    }
                  }
                }
              }
              frame #3 {
                # "Trigger \"start hyper\" event"
                n4897 = property on="Super Hidden" class="Bool (strict)"() -> ("Value"=w6353:bool)  [unwired: 2 in, 2 out]
                n4898 = property on="Super Hidden" class="Bool (strict)"("Val(Sgnl)"=w6353) -> ()  [unwired: 2 in, 2 out]
              }
            }
            n4899 = property on="Current SuperHyper Value" class="DigNum (strict)"("Value"=w6180) -> ()  [unwired: 2 in, 2 out]
          }
          frame True {
            # "When step values are all finished"
            n4900 = Enqueue Element(queue=w6359, element="Idle") -> ()  [unwired: 2 in, 3 out]
            n4901 = property on="Stop SuperHyper" class="Bool"("DisabledEnum"=T12."Disabled and Grayed Out" ("Disabled")) -> ()  [unwired: 2 in, 2 out]
            n4902 = property on="StartSuperHyper" class="Bool"("DisabledEnum"=T12."Enabled" ("Disabled")) -> ()  [unwired: 2 in, 2 out]
            n4903 = property on="Sweep Direction3" class="Str"("Value"="Finished!" ("Sweep Direction"), "Text.TextColor"=u32 16711680 ("Text.Text Colors:Text Color")) -> ()  [unwired: 2 in, 2 out]
          }
        }
      }
      frame "Quit" {
      }
    }
  }
  n4904 = while {
    tunnel: w3 -> [w6363]
    tunnel: w2 -> [w6361]
    tunnel: w1 -> [w6360]
    stop <- w6362 stop-if-true
    # "This loop is the producer loop."
    n4905 = event shown="[8] \"Populate step table?\": Value Change" {
      selector: _ -> [_ _ _ _ _ _ _ _ _ _ _ _ _ _ _ _ _ _ _ _ _ _ _ _ _ _ _]
      dyn-events: _ -> [_ _ _ _ _ _ _ _ _ _ _ _ _ _ _ _ _ _ _ _ _ _ _ _ _ _ _]
      timeout: _ -> [_ _ _ _ _ _ _ _ _ _ _ _ _ _ _ _ _ _ _ _ _ _ _ _ _ _ _]
      tunnel: w6363 -> [_ w6365 _ _ _ _ _ w6487 _ _ _ _ _ _ w6819 w6824 w6829 w6832 w6839 w6847 w6852 w6856 w6945 w6999 _ _ _]
      tunnel: [_ _ _ _ _ _ _ TRUE _ _ _ _ _ _ _ _ _ _ _ _ _ _ _ _ _ _ _] -> w6362
      tunnel: w6361 -> [_ _ _ _ _ _ _ _ _ _ _ _ _ _ _ _ _ _ _ _ _ _ _ _ _ w7057 _]
      tunnel: w6360 -> [_ _ _ _ _ _ _ _ _ _ _ _ _ _ _ _ _ _ _ _ _ _ _ _ _ _ w7082]
      event Timeout {
        n4906 = event-data() -> ()  [unwired: 1 in, 3 out]
      }
      event "Initialize": Value Change {
        n4907 = event-data() -> ()  [unwired: 1 in, 6 out]
        n4908 = Enqueue Element(queue=w6365, element="Idle") -> ()  [unwired: 2 in, 3 out]
      }
      event "Step Loop": Value Change {
        n4909 = event-data() -> ()  [unwired: 1 in, 1 out]
        n4910 = case shown="True" "Step Loop" {
          frame True {
            w6380 = T12."Enabled" ("Disabled")
            w6382 = T12."Disabled and Grayed Out" ("Disabled")
            n4911 = property on="Ramp\n Down" class="Bool"("DisabledEnum"=w6382) -> ()  [unwired: 2 in, 2 out]
            n4912 = property on="iTC_addr_sweep" class="VISAName"("DisabledEnum"=w6382) -> ()  [unwired: 2 in, 2 out]
            n4913 = property on="sweep" class="RadioBtnsControl (strict)"("DisabledEnum"=w6382) -> ()  [unwired: 2 in, 2 out]
            n4914 = property on="2182A 1 addr" class="DigNum (strict)"("DisabledEnum"=w6382) -> ()  [unwired: 2 in, 2 out]
            n4915 = property on="2182A 2 addr" class="DigNum (strict)"("DisabledEnum"=w6382) -> ()  [unwired: 2 in, 2 out]
            n4916 = property on="2182A 3 addr" class="DigNum (strict)"("DisabledEnum"=w6382) -> ()  [unwired: 2 in, 2 out]
            n4917 = property on="2182A 4 addr" class="DigNum (strict)"("DisabledEnum"=w6382) -> ()  [unwired: 2 in, 2 out]
            n4918 = property on="2400 1 addr" class="DigNum (strict)"("DisabledEnum"=w6382) -> ()  [unwired: 2 in, 2 out]
            n4919 = property on="iPS_addr_sweep" class="VISAName"("DisabledEnum"=w6382) -> ()  [unwired: 2 in, 2 out]
            n4920 = property on="Sweep Down" class="Bool"("DisabledEnum"=w6382) -> ()  [unwired: 2 in, 2 out]
            n4921 = property on="SR830 2 addr" class="DigNum (strict)"("DisabledEnum"=w6382) -> ()  [unwired: 2 in, 2 out]
            n4922 = property on="SR830 3 addr" class="DigNum (strict)"("DisabledEnum"=w6382) -> ()  [unwired: 2 in, 2 out]
            n4923 = property on="2400 2 addr" class="DigNum (strict)"("DisabledEnum"=w6382) -> ()  [unwired: 2 in, 2 out]
            n4924 = property on="2400 3 addr" class="DigNum (strict)"("DisabledEnum"=w6382) -> ()  [unwired: 2 in, 2 out]
            n4925 = property on="2336A addr" class="VISAName"("DisabledEnum"=w6382) -> ()  [unwired: 2 in, 2 out]
            n4926 = property on="SR830 1 addr" class="DigNum (strict)"("DisabledEnum"=w6382) -> ()  [unwired: 2 in, 2 out]
            n4927 = property on="SR830 4 addr" class="DigNum (strict)"("DisabledEnum"=w6382) -> ()  [unwired: 2 in, 2 out]
            n4928 = property on="Ramp \nUp" class="Bool"("DisabledEnum"=w6382) -> ()  [unwired: 2 in, 2 out]
            n4929 = property on="Sweep Up" class="Bool"("DisabledEnum"=w6382) -> ()  [unwired: 2 in, 2 out]
            n4930 = property on="Tolerance_Sweep" class="DigNum (strict)"("DisabledEnum"=w6382) -> ()  [unwired: 2 in, 2 out]
            n4931 = property on="Step and Hyerloop Setups" class="TabCtl (strict)"() -> ("Pages"=w6377:refnum<vi>[])  [unwired: 2 in, 2 out]
